vi "Door Access.vi"() -> ()   [LabVIEW 2014]
uses:
  Control 2.ctl
  <vilib>/userdefined/High Color/IMAQdx.ctl
  <vilib>/Instr/_visa.llb/VISA Configure Serial Port (Instr).vi
  <vilib>/vision/driver/NI_Vision_Acquisition_Software.lvlib
panel:
  out "path":path
  out "Intruder Photograph":T1(plugin-control)
  out "Status":string
  out "Password":string
  out "Log":string
  out "Read Mode":T2
  out "Not Match":bool
  out "CMD":string
  out "Card Num":string
  out "Match":bool
  in  "stop":bool
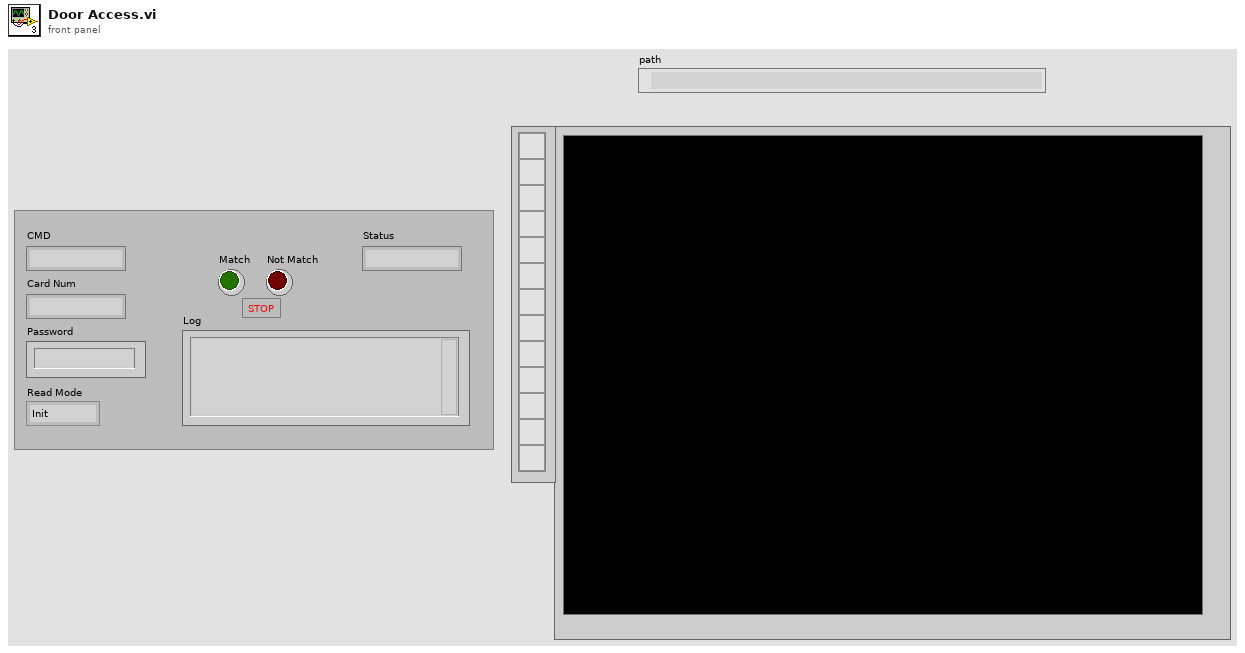
[diagram p1: front panel]
types:
  T1 = typedef "IMAQ Image.ctl" = refnum<image>
  T2 = typedef "Control 2.ctl" = enum16{"Init", "Get Cmd, Default", "Match", "Check Right", "Unmatch", "Timeout"}
  T3 = typedef "IMAQdx.ctl" = refnum<k21>
  T4 = enum16{"open", "replace", "create", "open or create", "replace or create", "replace or create with confirmation"}
  T5 = enum16{"Init", "Get Cmd, Default", "Match", "Check Right", "Unmatch", "Timeout"}
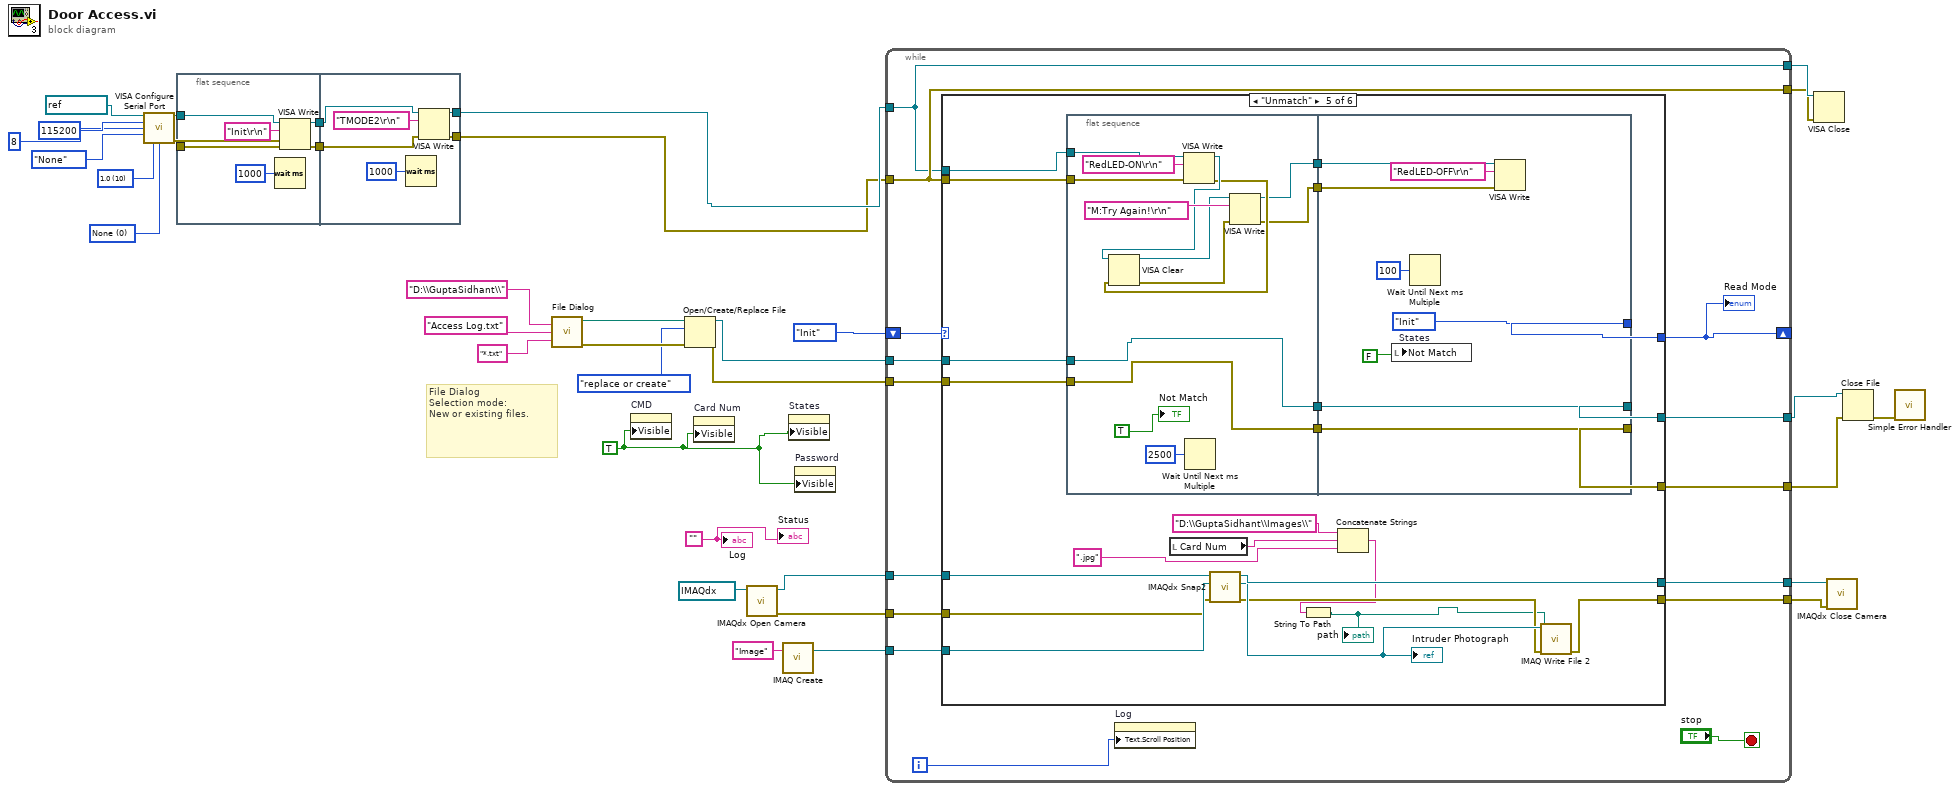
[diagram p0: block diagram]
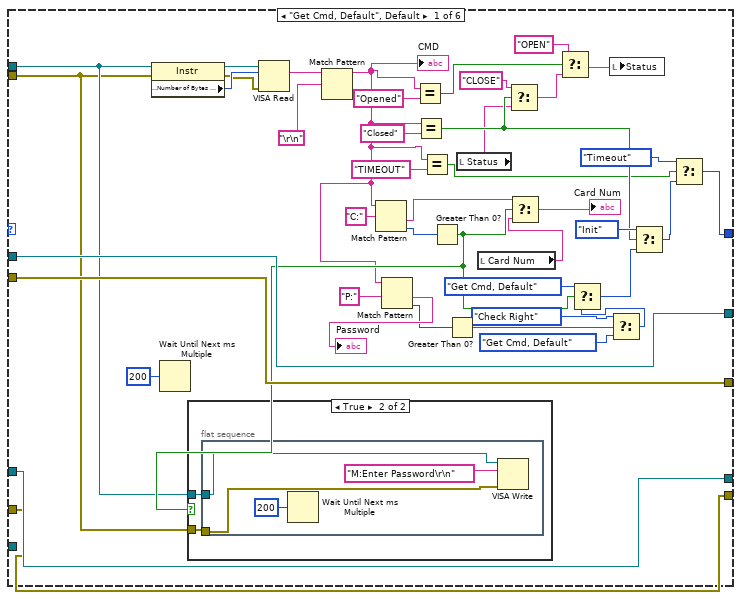
[diagram p2: hidden frame]
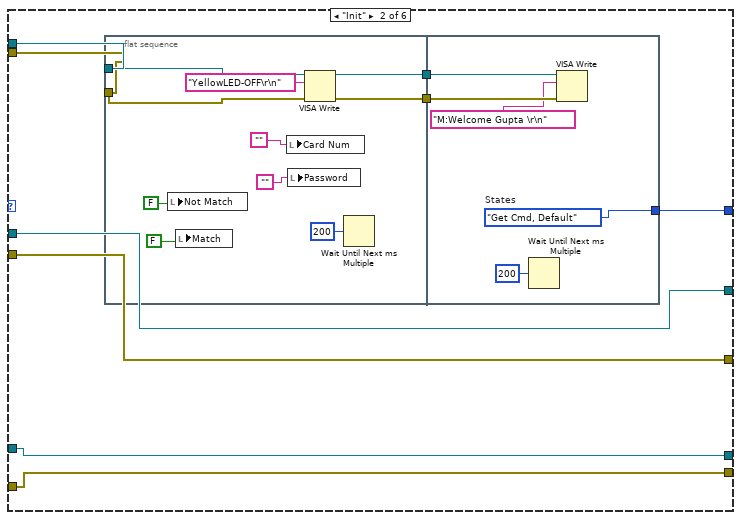
[diagram p4: hidden frame]
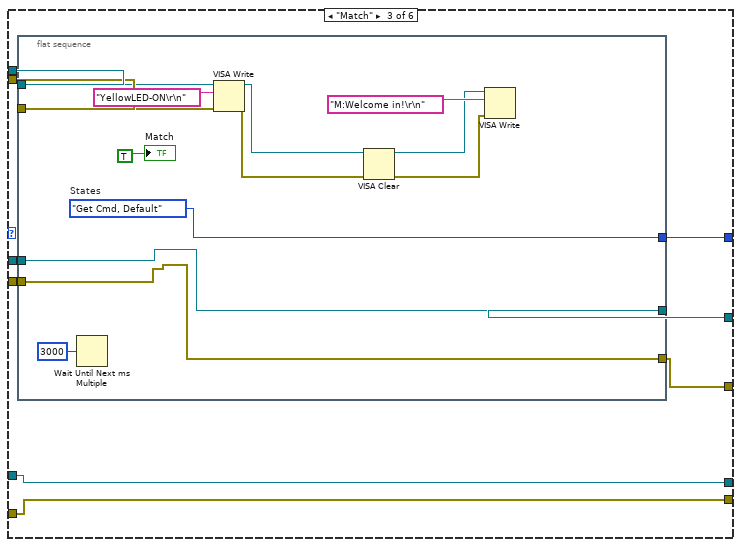
[diagram p5: hidden frame]
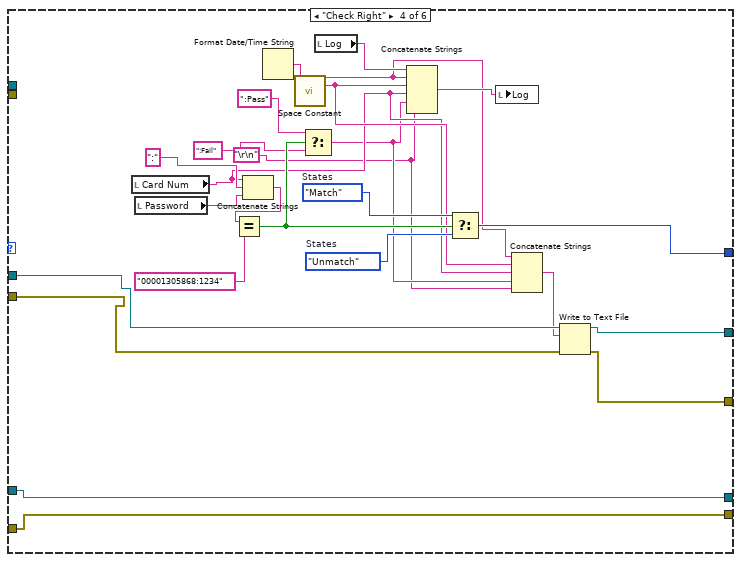
[diagram p6: hidden frame]
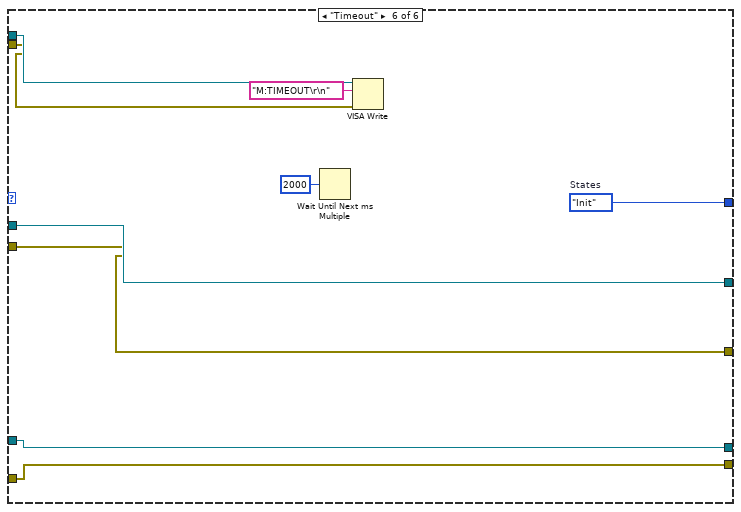
[diagram p7: hidden frame]
diagram:
  w10 = ""
  w11 = TRUE
  w30 = u16 0 items=["None", "XON/XOFF", "RTS/CTS", "XON/XOFF & RTS/CTS", "DTR/DSR", "XON/XOFF & DTR/DSR"] ("flow control (0:none)")
  w31 = u16 10 items=["1.0"=10, "1.5"=15, "2.0"=20] ("stop bits (10: 1 bit)")
  # "File Dialog\nSelection mode:\nNew or existing files."
  n1 = call-poly "VISA Configure Serial Port"("VISA resource name"=refnum<visa-resource-name> "COM4", "baud rate (9600)"=u32 115200, "data bits (8)"=u16 8, "parity (0:none)"=enum16{"None", "Odd", "Even", "Mark", "Space"}."None", "stop bits (10: 1 bit)"=w31, "flow control (0:none)"=w30) -> ("VISA resource name out"=w29:refnum<visa-resource-name>, "error out"=w28:errorcluster)  [unwired: 8 in]
  n2 = flat-sequence {
    tunnel: w29 -> [w39]
    tunnel: w28 -> [w38]
    tunnel: [w37] -> w27
    tunnel: [w36] -> w26
    tunnel: w27 -> [w45]
    tunnel: w26 -> [w44]
    tunnel: [w43] -> w9
    tunnel: [w42] -> w8
    frame #0 {
      n3 = Wait (ms)(milliseconds to wait=u32 1000) -> ()  [unwired: 1 out]
      n4 = VISA Write(VISA resource name=w39, write buffer="Init\r\n", error in (no error)=w38) -> (VISA resource name out=w37:refnum<visa-resource-name>, error out=w36:errorcluster)  [unwired: 1 out]
    }
    frame #1 {
      n5 = Wait (ms)(milliseconds to wait=u32 1000) -> ()  [unwired: 1 out]
      n6 = VISA Write(VISA resource name=w45, write buffer="TMODE2\r\n", error in (no error)=w44) -> (VISA resource name out=w43:refnum<visa-resource-name>, error out=w42:errorcluster)  [unwired: 1 out]
    }
  }
  n7 = call "File Dialog"("prompt"="D:\\GuptaSidhant\\", "default name"="Access Log.txt", "pattern (all files)"="*.txt" ("pattern label")) -> ("selected path"=w18:path, "error out"=w19:errorcluster)  [unwired: 9 in, 2 out]
  n8 = property on="CMD" class="Str"("Visible"=w11) -> ()  [unwired: 2 in, 2 out]
  n9 = Open/Create/Replace File(file path (use dialog)=w18, error in=w19, operation (0:open)=T4."replace or create") -> (refnum out=w16:refnum<file>, error out=w15:errorcluster)  [unwired: 3 in, 1 out]
  n10 = property on="Card Num" class="Str"("Visible"=w11) -> ()  [unwired: 2 in, 2 out]
  n11 = call <vilib>:"IMAQdx Open Camera.vi"("Session In"=T3 "cam0") -> ("error out"=w3:errorcluster, "Session Out"=w4:T3)  [unwired: 9 in]
  n12 = call "IMAQ Create"("Image Name"="Image") -> ("New Image"=w5:T1)  [unwired: 4 in, 1 out]
  n13 = property on="States" class="Enum (strict)"("Visible"=w11) -> ()  [unwired: 2 in, 2 out]
  n14 = property on="Password" class="Str"("Visible"=w11) -> ()  [unwired: 2 in, 2 out]
  n15 = while {
    tunnel: [w59] -> w25
    tunnel: w9 -> [w59]
    shift-right: [w58] -> _
    shift-left: Control_2."Init" ("States") -> [w61]
    tunnel: w8 -> [w60]
    tunnel: [w60] -> w23
    tunnel: w16 -> [w57]
    tunnel: w15 -> [w56]
    tunnel: [w55] -> w14
    tunnel: [w54] -> w13
    tunnel: w5 -> [w52]
    tunnel: w4 -> [w51]
    tunnel: w3 -> [w50]
    tunnel: [w49] -> w2
    tunnel: [w48] -> w1
    i -> [w53]
    stop <- "stop" stop-if-true
    n16 = case shown="\"Unmatch\"" w61 {
      tunnel: w60 -> [w71 w116 w138 _ w196 w231]
      tunnel: [w65 w120 w144 w179 w204 w235] -> w58
      tunnel: w59 -> [w72 w117 w139 _ w197 w232]
      tunnel: w57 -> [w94 w119 w143 w170 w203 w234]
      tunnel: w56 -> [w93 w118 w142 w167 w202 w233]
      tunnel: [w94 w119 w141 w169 w198 w234] -> w55
      tunnel: [w93 w118 w140 w168 w200 w233] -> w54
      tunnel: w52 -> [_ _ _ _ w193 _]
      tunnel: w51 -> [w64 w113 w137 w159 w192 w228]
      tunnel: w50 -> [w63 w112 w136 w158 w191 w227]
      tunnel: [w64 w113 w137 w159 w190 w228] -> w49
      tunnel: [w63 w112 w136 w158 w187 w227] -> w48
      frame "Get Cmd, Default", Default {
        n17 = property class="Instr"(reference=w72, error in=w71) -> (reference out=w103:refnum<visa-resource-name>, error out=w102:errorcluster, "Serial Settings:Number of Bytes at Serial Port"=w104:u32)
        n18 = Wait Until Next ms Multiple(millisecond multiple=u32 200) -> ()  [unwired: 1 out]
        n19 = VISA Read(VISA resource name=w103, byte count=w104, error in (no error)=w102) -> (read buffer=w99:string)  [unwired: 3 out]
        n20 = Match Pattern(string=w99, regular expression="\r\n") -> (before substring=w70:string)  [unwired: 1 in, 3 out]
        "CMD" <- w70
        n21 = Match Pattern(string=w70, regular expression="C:") -> (after substring=w100:string, offset past match=w76:i32)  [unwired: 1 in, 2 out]
        n22 = Match Pattern(string=w70, regular expression="P:") -> (after substring=→"Password":string, offset past match=w75:i32)  [unwired: 1 in, 2 out]
        n23 = Equal?(x=w70, y="Opened") -> (x = y?=w80:bool)
        n24 = Equal?(x=w70, y="Closed") -> (x = y?=w81:bool)
        n25 = Equal?(x=w70, y="TIMEOUT") -> (x = y?=w68:bool)
        n26 = Greater Than 0?(x=w76) -> (x > 0?=w73:bool)
        n27 = case shown="True" w73 {
          tunnel: w72 -> [_ w107]
          tunnel: w71 -> [_ w106]
          frame False {
          }
          frame True {
            n28 = flat-sequence {
              tunnel: w107 -> [w110]
              tunnel: w106 -> [w109]
              frame #0 {
                n29 = Wait Until Next ms Multiple(millisecond multiple=u32 200) -> ()  [unwired: 1 out]
                n30 = VISA Write(VISA resource name=w110, write buffer="M:Enter Password\r\n", error in (no error)=w109) -> ()  [unwired: 3 out]
              }
            }
          }
        }
        n31 = Greater Than 0?(x=w75) -> (x > 0?=w90:bool)
        n32 = local read "Status"() -> (w78:string)
        n33 = local read "Card Num"() -> (w97:string)
        n34 = Select(t="CLOSE", s=w81, f=w78) -> (s? t:f=w84:string)
        n35 = Select(t=w100, s=w73, f=w97) -> (s? t:f=→"Card Num":string)
        n36 = Select(t="OPEN", s=w80, f=w84) -> (s? t:f=w83:string)
        n37 = local write "Status"(w83) -> ()
        n38 = Select(t=T5."Check Right" ("States"), s=w90, f=T5."Get Cmd, Default" ("States")) -> (s? t:f=w89:T5)
        n39 = Select(t=T5."Get Cmd, Default" ("States"), s=w73, f=w89) -> (s? t:f=w74:T5)
        n40 = Select(t=T5."Init", s=w81, f=w74) -> (s? t:f=w66:T5)
        n41 = Select(t=Control_2."Timeout" ("States"), s=w68, f=w66) -> (s? t:f=w65:T2)
      }
      frame "Init" {
        n42 = flat-sequence {
          tunnel: w117 -> [w125]
          tunnel: w116 -> [w126]
          tunnel: [w123] -> w115
          tunnel: [w122] -> w114
          tunnel: [w132] -> w120
          tunnel: w115 -> [w135]
          tunnel: w114 -> [w134]
          frame #0 {
            n43 = local write "Not Match"(FALSE) -> ()
            n44 = local write "Match"(FALSE) -> ()
            n45 = local write "Card Num"("") -> ()
            n46 = local write "Password"("") -> ()
            n47 = VISA Write(VISA resource name=w125, write buffer="YellowLED-OFF\r\n", error in (no error)=w126) -> (VISA resource name out=w123:refnum<visa-resource-name>, error out=w122:errorcluster)  [unwired: 1 out]
            n48 = Wait Until Next ms Multiple(millisecond multiple=u32 200) -> ()  [unwired: 1 out]
          }
          frame #1 {
            w132 = T5."Get Cmd, Default"  # States
            n49 = Wait Until Next ms Multiple(millisecond multiple=u32 200) -> ()  [unwired: 1 out]
            n50 = VISA Write(VISA resource name=w135, write buffer="M:Welcome Gupta \r\n", error in (no error)=w134) -> ()  [unwired: 3 out]
          }
        }
      }
      frame "Match" {
        n51 = flat-sequence {
          tunnel: w143 -> [w154]
          tunnel: w142 -> [w153]
          tunnel: w139 -> [w152]
          tunnel: w138 -> [w151]
          tunnel: [w154] -> w141
          tunnel: [w153] -> w140
          tunnel: [w150] -> w144
          frame #0 {
            w150 = T5."Get Cmd, Default"  # States
            n52 = Wait Until Next ms Multiple(millisecond multiple=u32 3000) -> ()  [unwired: 1 out]
            n53 = VISA Write(VISA resource name=w152, write buffer="YellowLED-ON\r\n", error in (no error)=w151) -> (VISA resource name out=w148:refnum<visa-resource-name>, error out=w145:errorcluster)  [unwired: 1 out]
            n54 = VISA Clear(VISA resource name=w148, error in (no error)=w145) -> (VISA resource name out=w147:refnum<visa-resource-name>, error out=w146:errorcluster)
            n55 = VISA Write(VISA resource name=w147, write buffer="M:Welcome in!\r\n", error in (no error)=w146) -> ()  [unwired: 3 out]
            "Match" <- TRUE
          }
        }
      }
      frame "Check Right" {
        w161 = "\r\n"
        w180 = T5."Unmatch"  # States
        w181 = T5."Match"  # States
        n56 = local read "Card Num"() -> (w163:string)
        n57 = local read "Password"() -> (w172:string)
        n58 = Concatenate Strings(w163, ":", w172) -> (w171:string)
        n59 = Equal?(x=w171, y="00001305868:1234") -> (x = y?=w176:bool)
        n60 = Format Date/Time String() -> (date/time string=w165:string)  [unwired: 3 in]
        n61 = call <vilib>:"Space Constant.vi"() -> ("String"=w164:string)
        n62 = Select(t=":Pass", s=w176, f=":Fail") -> (s? t:f=w162:string)
        n63 = local read "Log"() -> (w177:string)
        n64 = Concatenate Strings(w177, w165, w164, w163, w162, w161) -> (w166:string)
        n65 = Select(t=w181, s=w176, f=w180) -> (s? t:f=w179:T5)
        n66 = local write "Log"(w166) -> ()
        n67 = Concatenate Strings(w165, w164, w163, w162, w161) -> (w160:string)
        n68 = Write to Text File(file (use dialog)=w170, text=w160, error in=w167) -> (refnum out=w169:refnum<file>, error out=w168:errorcluster)  [unwired: 1 in, 1 out]
      }
      frame "Unmatch" {
        n69 = flat-sequence {
          tunnel: w203 -> [w213]
          tunnel: w202 -> [w212]
          tunnel: [w212] -> w201
          tunnel: [w213] -> w199
          tunnel: w197 -> [w216]
          tunnel: w196 -> [w215]
          tunnel: [w206] -> w195
          tunnel: [w205] -> w194
          tunnel: [w225] -> w204
          tunnel: [w223] -> w200
          tunnel: w201 -> [w223]
          tunnel: [w222] -> w198
          tunnel: w199 -> [w222]
          tunnel: w195 -> [w221]
          tunnel: w194 -> [w220]
          frame #0 {
            n70 = VISA Write(VISA resource name=w216, write buffer="RedLED-ON\r\n", error in (no error)=w215) -> (VISA resource name out=w208:refnum<visa-resource-name>, error out=w207:errorcluster)  [unwired: 1 out]
            n71 = VISA Clear(VISA resource name=w208, error in (no error)=w207) -> (VISA resource name out=w210:refnum<visa-resource-name>, error out=w209:errorcluster)
            n72 = Wait Until Next ms Multiple(millisecond multiple=u32 2500) -> ()  [unwired: 1 out]
            n73 = VISA Write(VISA resource name=w210, write buffer="M:Try Again!\r\n", error in (no error)=w209) -> (VISA resource name out=w206:refnum<visa-resource-name>, error out=w205:errorcluster)  [unwired: 1 out]
            "Not Match" <- TRUE
          }
          frame #1 {
            w225 = T5."Init"  # States
            n74 = local write "Not Match"(FALSE) -> ()
            n75 = Wait Until Next ms Multiple(millisecond multiple=u32 100) -> ()  [unwired: 1 out]
            n76 = VISA Write(VISA resource name=w221, write buffer="RedLED-OFF\r\n", error in (no error)=w220) -> ()  [unwired: 3 out]
          }
        }
        n77 = local read "Card Num"() -> (w185:string)
        n78 = call <vilib>:"IMAQdx Snap2.vi"("error in"=w191, "Image In"=w193, "Session In"=w192) -> ("error out"=w188:errorcluster, "Image Out"=w189:T1, "Session Out"=w190:T3)  [unwired: 6 in]
        "Intruder Photograph" <- w189
        n79 = Concatenate Strings("D:\\GuptaSidhant\\Images\\", w185, ".jpg") -> (w183:string)
        n80 = String To Path(string=w183) -> (path=w184:path)
        "path" <- w184
        n81 = call-poly "IMAQ Write File 2"("error in (no error)"=w188, "File Path"=w184, "Image"=w189) -> ("error out"=w187:errorcluster)  [unwired: 7 in, 1 out]
      }
      frame "Timeout" {
        w235 = T5."Init"  # States
        n82 = Wait Until Next ms Multiple(millisecond multiple=u32 2000) -> ()  [unwired: 1 out]
        n83 = VISA Write(VISA resource name=w232, write buffer="M:TIMEOUT\r\n", error in (no error)=w231) -> ()  [unwired: 3 out]
      }
    }
    "Read Mode" <- w58
    n84 = property on="Log" class="Str"("Text.Scroll Position"=w53) -> ()  [unwired: 2 in, 2 out]
  }
  n85 = VISA Close(VISA resource name=w25, error in (no error)=w23) -> ()  [unwired: 1 out]
  n86 = call <vilib>:"IMAQdx Close Camera.vi"("error in"=w1, "Session In"=w2) -> ()  [unwired: 9 in, 1 out]
  n87 = Close File(refnum=w14, error in=w13) -> (error out=w17:errorcluster)  [unwired: 1 out]
  n88 = call <vilib>:"Simple Error Handler.vi"("error in (no error)"=w17) -> ()  [unwired: 4 in, 5 out]
  "Log" <- w10
  "Status" <- w10
